vi "Motor Multiplexer-Dual.vi"() -> ()   [LabVIEW 2009]
uses:
  <vilib>/NXT/Block Support/NXT_InputPort.ctl
  <vilib>/NXT/Subs/LVHSConnector.ctl
  mindsensors.com LVEE Toolkit/Dual/Motor Multiplexer-DM.vi
panel:
  in  "stop":bool
  out "Status":bool
  in  "Input of Motor Multiplexer":T1={"Mode"=1, "Direction"=FALSE, "Motor"=1, "Power"=100} {"Power" max=100 step=1; "Motor" min=1 max=4 step=1; "Mode" items=["RUN", "FLT", "BRK"]}
  out "NXT dup":T2 caption="NXT"
  in  "NXT":T2
  in  "Input Port":T3 items=["Port 1", "Port 2", "Port 3", "Port 4"]
  # "mindsensors.com\nCopyright (c) 2009 by mindsensors.com\nEmail: info (<at>) mindsensors (<dot>) com\n\nThis program is free software. You can redistribute it and/or modify\nit under the terms of the GNU General Public License as published by\nthe Free Software Foundation; version 3 of the License.\nRead the license at: http://www.gnu.org/licenses/gpl.txt"
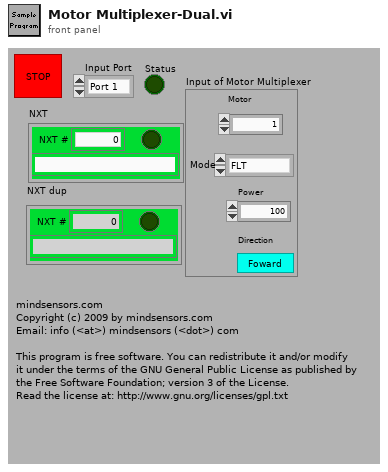
[diagram p1: front panel]
types:
  T1 = cluster{"Mode":u8, "Direction":bool, "Motor":u8, "Power":u8}
  T2 = typedef "LVHSConnector.ctl" = cluster{"error":errorcluster, "address":string, "NXT #":i32, "Show Error":bool}
  T3 = typedef "NXT_InputPort.ctl" = u8
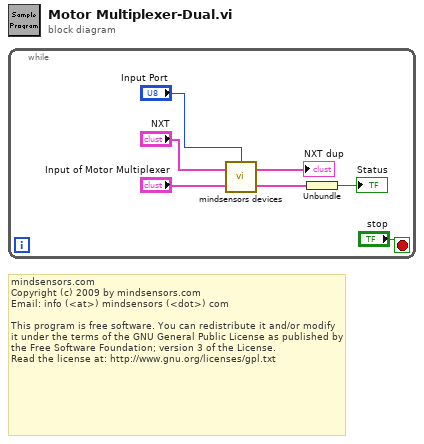
[diagram p0: block diagram]
diagram:
  # "mindsensors.com\nCopyright (c) 2009 by mindsensors.com\nEmail: info (<at>) mindsensors (<dot>) com\n\nThis program is free software. You can redistribute it and/or modify\nit under the terms of the GNU General Public License as published by\nthe Free Software Foundation; version 3 of the License.\nRead the license at: http://www.gnu.org/licenses/gpl.txt"
  n1 = while {
    stop <- "stop" stop-if-true
    n2 = call-poly "mindsensors devices.vi"("Input of Motor Multiplexer"="Input of Motor Multiplexer", "NXT"="NXT", "Input Port"="Input Port") -> ("Output of Motor Multiplexer"=w3:cluster{"Status":bool}, "NXT dup"=→"NXT dup":T2)
    n3 = Unbundle(w3) -> ("Status"=→"Status":bool)
  }
